vi "Read Max clients.vi"(8 "error in (no error)":errorcluster, 11 "Server in":refnum<class "SLMServer.lvclass">) -> (0 "error out":errorcluster, 2 "Max clients":T2(array[cluster]), 3 "Server out":refnum<class "SLMServer.lvclass">)   [LabVIEW 2013, in "SLMServer.lvlib" / "SLMServer.lvclass"]
uses:
  SLMServer.lvclass
  Supported-module-types.ctl
  SLMServer.lvclass/SLMServer.ctl
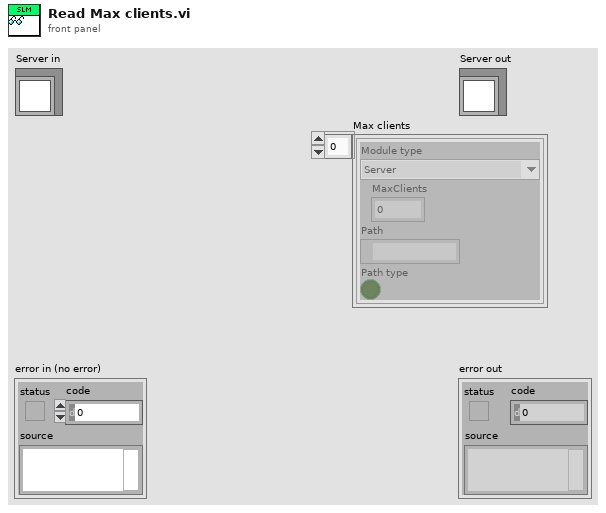
[diagram p1: front panel]
types:
  T1 = typedef "SLMServer.lvlib/SLMServer.lvclass/Supported-module-types.ctl" = enum16{"SLMControl", "PowderDeposition", "CameraVision", "Server", "All", "StrategyParser", "MaterialCharacterization", "StatusMonitor", "SLMSimulation", "LaserCharacterization"}
  T2 = cluster{"Module type":T1, "MaxClients":i32, "Path":path, "Path type":bool}[]
  T3 = cluster{"Module type":T1, "MaxClients":i32, "Path":path, "Relative path?":bool}[]
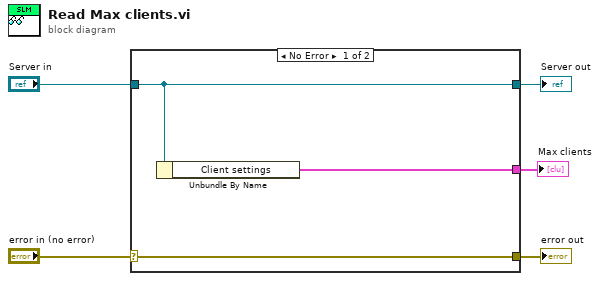
[diagram p0: block diagram]
diagram:
  n1 = case shown="No Error" "error in (no error)" {
    selector: "error in (no error)" -> [w8 w9]
    tunnel: [w8 w9] -> w4
    tunnel: [w7 w10] -> w2
    tunnel: "Server in" -> [w7 w10]
    tunnel: [w6 _] -> w1
    frame No Error {
      n2 = Unbundle By Name(w7) -> ("Client settings"=w6:T3)
    }
    frame Error {
    }
  }
  "error out" <- w4
  "Server out" <- w2
  "Max clients" <- w1
